vi "close mb.vi"(8 "error in (no error)":errorcluster) -> (0 "error out":errorcluster)   [LabVIEW 2016, in "超标留样集成.lvlib" / "DR803M4.lvlib"]
uses:
  DR803M4.lvlib
  Global variable/input variable.vi
  <vilib>/Plasmionique/MB Master/MB_Master_Serial/MB_Master_Serial.lvclass
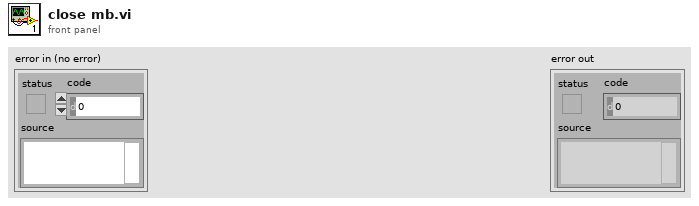
[diagram p1: front panel]
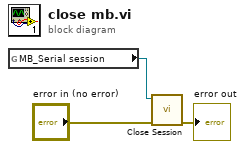
[diagram p0: block diagram]
diagram:
  n1 = global read "input variable.vi" "MB_Serial session"() -> (w3:refnum<class "MB_Master_Serial.lvclass">)
  n2 = call-dynamic "Close Session.vi"("error in (no error)"="error in (no error)", "MB_Serial session"=w3) -> ("error out"=→"error out":errorcluster)  [unwired: 9 in]
